vi "データポインタ経由の画像操作テスト(.NET).vi"() -> ()   [LabVIEW 2020]
uses:
  DLL/VisionMemoryWatch/VisionMemoryWatch/bin/Debug/VisionMemoryWatch.dll
panel:
  out "Image Pixels (U8) 2":u8[][](array[numeric])
  in  "Image Pixels (U8) in":u8[][](array[numeric])=[[1, 2, 3, 4], [5, 6, 7, 8], [9, 10, 11, 12], [13, 14, 15, 16]]
  out "Image Pixels (U8)":u8[][](array[numeric])
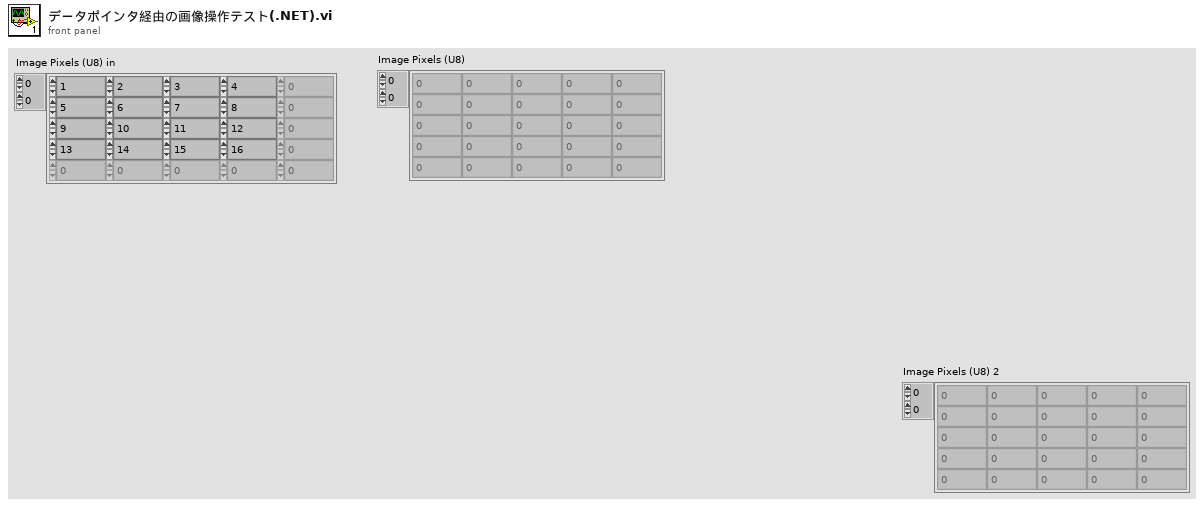
[diagram p1: front panel]
types:
  T1 = enum32{"Map Pixel Pointer", "Unmap Pixel Pointer", "Get Pixels Infos"}
  T2 = typedef "Image Type" = u32
  T3 = typedef "IMAQ Image.ctl" = refnum<image>
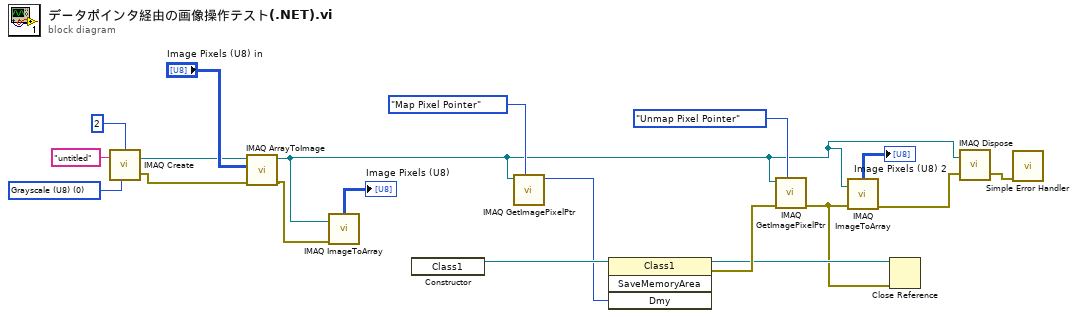
[diagram p0: block diagram]
diagram:
  w17 = T2 0 items=["Grayscale (U8)", "Grayscale (I16)", "Grayscale (SGL)", "Complex (CSG)", "RGB (U32)", "HSL (U32)", "RGB (U64)", "Grayscale (U16)"] ("Image Type")
  n1 = call "IMAQ Create"("Border Size"=2, "Image Name"="untitled", "Image Type"=w17) -> ("New Image"=w12:T3, "error out"=w11:errorcluster)  [unwired: 2 in]
  n2 = call "IMAQ ArrayToImage"("error in (no error)"=w11, "Image Pixels (U8)"="Image Pixels (U8) in", "Image"=w12) -> ("error out"=w13:errorcluster, "Image Out"=w3:T3)  [unwired: 7 in]
  n3 = call "IMAQ ImageToArray"("error in (no error)"=w13, "Image"=w3) -> ("Image Pixels (U8)"=→"Image Pixels (U8)":u8[][])  [unwired: 2 in, 4 out]
  n4 = constructor class="Class1"() -> (reference out=w9:refnum<k24>)  [unwired: 3 in, 2 out]
  n5 = call "IMAQ GetImagePixelPtr"("Function"=T1."Map Pixel Pointer", "Image"=w3) -> ("Pixel Pointer out"=w8:u64)  [unwired: 4 in, 5 out]
  n6 = invoke class="Class1" method="SaveMemoryArea"(reference=w9, "Dmy"=w8) -> (reference out=w6:refnum<k24>, error out=w7:errorcluster)  [unwired: 2 in, 2 out]
  n7 = call "IMAQ GetImagePixelPtr"("Function"=T1."Unmap Pixel Pointer", "error in (no error)"=w7, "Image"=w3) -> ("error out"=w2:errorcluster)  [unwired: 3 in, 5 out]
  n8 = call "IMAQ ImageToArray"("error in (no error)"=w2, "Image"=w3) -> ("error out"=w1:errorcluster, "Image Pixels (U8)"=→"Image Pixels (U8) 2":u8[][])  [unwired: 2 in, 3 out]
  n9 = Close Reference(reference=w6, error in (no error)=w2) -> ()  [unwired: 1 out]
  n10 = call "IMAQ Dispose"("Image"=w3, "error in (no error)"=w1) -> ("error out"=w15:errorcluster)  [unwired: 4 in]
  n11 = call <vilib>:"Simple Error Handler.vi"("error in (no error)"=w15) -> ()  [unwired: 4 in, 5 out]
